vi "Trig port tester.vi"() -> ()   [LabVIEW 2017]
uses:
  <vilib>/rvi/eio/common/nirviEmuTemplateMethod_errors.vi
  <vilib>/rvi/Emulation/niFpgaGetClockAttributes.vi
  <vilib>/rvi/Emulation/niFpgaSctlEmulationGetInTimedLoop.vi
  <vilib>/rvi/Emulation/niFpgaEmulationReportErrorSimple.vi
  <vilib>/rvi/Emulation/niFpgaProcessEmulError.vi
  <vilib>/rvi/Emulation/niFpgaCriticalErrorInLSC.vi
  <vilib>/eio/EIONode/EIONode.xnode
panel:
  in  "stop":bool
  out "IO Module\\Initialization Done":bool
  out "Boolean 2":bool
  in  "Boolean":bool
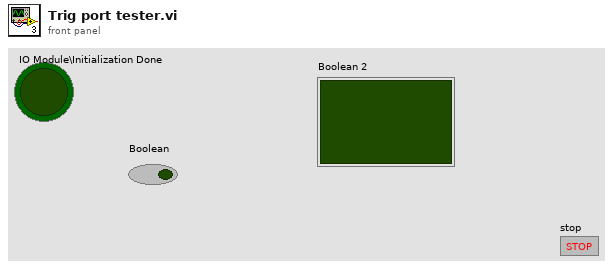
[diagram p1: front panel]
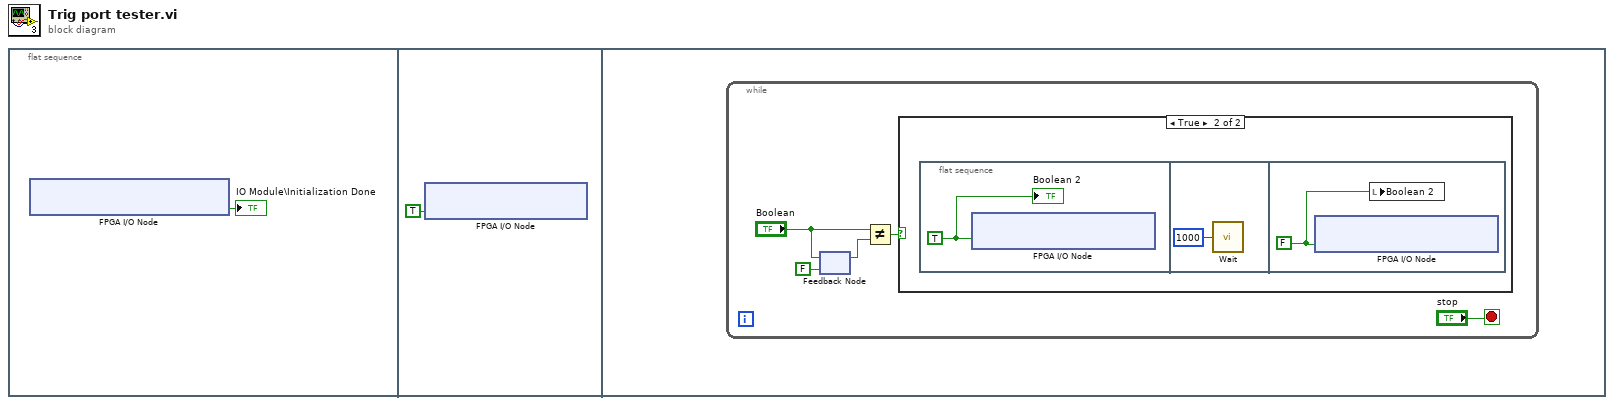
[diagram p0: block diagram]
diagram:
  n1 = flat-sequence {
    frame #0 {
      n2 = xnode "FPGA I/O Node"() -> ("IO Module\\Initialization Done"=→"IO Module\\Initialization Done":bool)  [unwired: 1 in, 1 out]
    }
    frame #1 {
      n3 = xnode "FPGA I/O Node"("IO Module\\Trigger WE"=TRUE ("IO Module\\Trigger WE")) -> ()  [unwired: 1 in, 1 out]
    }
    frame #2 {
      n4 = while "Timed Loop" {
        stop <- "stop" stop-if-true
        n5 = feedback #1(FALSE ("Boolean")) -> (w6:bool)
        n6 = feedback-in #1("Boolean") -> ()
        n7 = Not Equal?(x="Boolean", y=w6) -> (x != y?=w5:bool)
        n8 = case shown="True" w5 {
          frame False {
          }
          frame True {
            n9 = flat-sequence {
              frame #0 {
                w8 = TRUE ("IO Module\\Trigger Output")
                n10 = xnode "FPGA I/O Node"("IO Module\\Trigger Output"=w8) -> ()  [unwired: 1 in, 1 out]
                "Boolean 2" <- w8
              }
              frame #1 {
                n11 = call "Wait"("Count(uSec)"=u32 1000) -> ()  [unwired: 1 out]
              }
              frame #2 {
                w10 = FALSE ("IO Module\\Trigger Output")
                n12 = xnode "FPGA I/O Node"("IO Module\\Trigger Output"=w10) -> ()  [unwired: 1 in, 1 out]
                n13 = local write "Boolean 2"(w10) -> ()
              }
            }
          }
        }
      }
    }
  }
